vi "AE_continuousread.vi"() -> ()   [LabVIEW 2012]
doc: "I. Description:\nThis example demonstrates how to continuously acquire unscaled and save the data in a binary file. You can use the Graph Acquired Binary Data.VI to read and plot the scaled data on a Waveform Graph.\n\nII. Instructions for Running:\n1. Select the physical channel to correspond to where your signal is input on the DAQ device.\n2. Enter the minimum and maximum voltage ranges.\nNote: For better accuracy try to match the input range to the expected voltage level of the measured signal.\n3. Set the rate of the acquisition Also set the Samples to Read control. This will determine how many samples are read each time the while loop iterates. This also determines how many points are plotted on the graph each iteration.\nNote: The rate should be at least twice as fast as the maximum frequency component of the signal being acquired.\n4. Select the File Properties. If the file path is left empty, it will bring up a dialog box to let you browse to the file. \n\nIII. Block Diagram Steps:\n1. Create or replace a file to store the data.\n2. Create an analog input voltage channel.\n3. Set the rate for the sample clock. Additionally, define the sample mode to be continuous.\n4. Create a header and write it to the binary file.\n5. Call the Start VI to start acquiring samples. \n6. Read the unscaled data in a loop until the user hits the stop button or an error occurs.\nNote: This example uses unscaled I32 reads. Some devices support unscaled reads in smaller widths, such as I16. To get the maximum performance out of your device, use the unscaled read with the smallest supported width.\n7. Transpose the unscaled array of data and append it to the file.\n8. Close the File.\n9. Call the Stop VI to stop acquiring samples.\n10. Use the popup dialog box to display an error if any.\n\nIV. I/O Connections Overview:\nMake sure your signal input terminal matches the Physical Channel I/O control. For further connection information, refer to your hardware reference manual."
uses:
  <vilib>/Utility/error.llb/DialogType.ctl
  <vilib>/DAQmx/read.llb/DAQmx Read (Analog 1D Wfm NChan NSamp).vi
  <vilib>/DAQmx/create/channels.llb/DAQmx Create Channel (AI-Voltage-Basic).vi
  <vilib>/DAQmx/configure/timing.llb/DAQmx Timing (Sample Clock).vi
  Instance          10 57Saved   Cont Acq&Graph Voltage - Write Data to File (CSV) .vi
  <vilib>/DAQmx/miscellaneous.llb/DAQmx Fill In Error Info.vi
panel:
  in  "Gain":u16(ring)=1 items=["20 dB", "40 dB", "60 dB"]
  in  "Test Name":string="test"
  in  "Storage Directory":path=path "C:/Users/User/Desktop/Users_2013-2014/Michael Rossol"
  in  "stop":bool
  in  "Physical Channel":tag="Dev1/ai0"
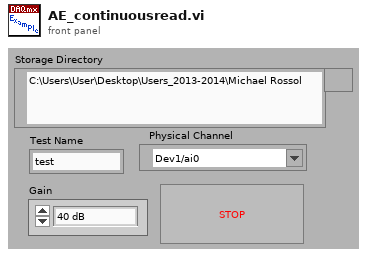
[diagram p1: front panel]
types:
  T1 = enum16{"open", "replace", "create", "open or create", "replace or create", "replace or create with confirmation"}
  T2 = typedef "DialogType.ctl" = u16
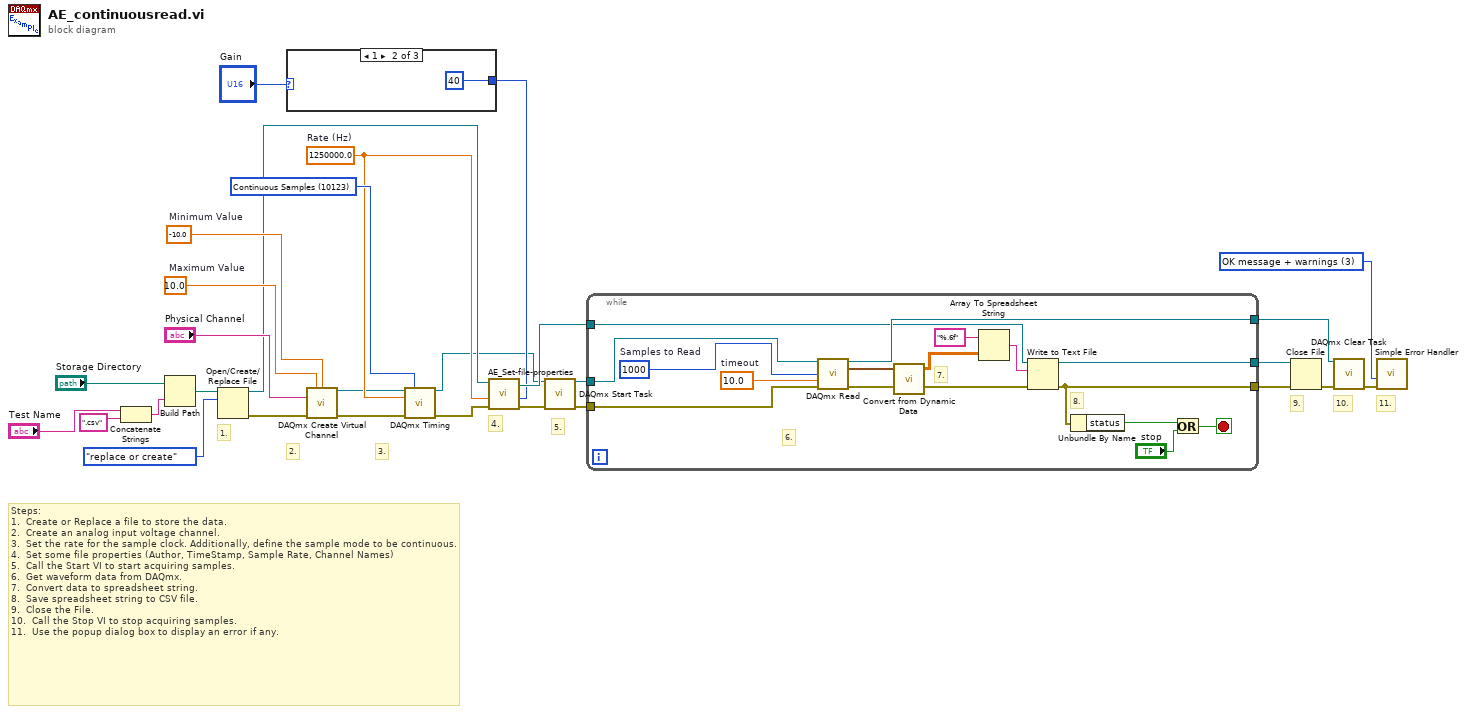
[diagram p0: block diagram]
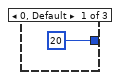
[diagram p2: hidden frame]
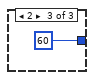
[diagram p3: hidden frame]
diagram:
  w13 = 1250000.0  # Rate (Hz)
  w28 = 10.0  # Maximum Value
  w29 = -10.0  # Minimum Value
  w19 = T2 3 items=["no dialog", "OK message", "continue or stop message", "OK message + warnings", "continue/stop + warnings"] ("type of dialog (OK msg:1)")
  w22 = 10123 items=["Finite Samples"=10178, "Continuous Samples"=10123] ("sample mode")
  # "11."
  # "10."
  # "4."
  # "9."
  # "3."
  # "5."
  # "Steps: \n1.  Create or Replace a file to store the data.\n2.  Create an analog input voltage channel.\n3.  Set the rate for the sample clock. Additionally, define the sample mode to be continuous.\n4.  Set some file properties (Author, TimeStamp, Sample Rate, Channel Names)\n5.  Call the Start VI to start acquiring samples.  \n6.  Get waveform data from DAQmx.\n7.  Convert data to spreadsheet string.\n8.  Save spreadsheet string to CSV file. \n9.  Close the File.\n10.  Call the Stop VI to stop acquiring samples.\n11.  Use the popup dialog box to display an error if any."
  # "2."
  # "1."
  n1 = Concatenate Strings("Test Name", ".csv" ("string")) -> (w6:string)
  n2 = Build Path(base path="Storage Directory", name or relative path=w6) -> (appended path=w4:path)
  n3 = Open/Create/Replace File(file path (use dialog)=w4, operation (0:open)=T1."replace or create") -> (refnum out=w10:refnum<file>, error out=w17:errorcluster)  [unwired: 4 in, 1 out]
  n4 = case shown="1" "Gain" {
    tunnel: [20 40 60] -> w2
    frame 0, Default {
    }
    frame 1 {
    }
    frame 2 {
    }
  }
  n5 = call-poly <vilib>:"DAQmx Create Virtual Channel.vi"("maximum value"=w28, "minimum value"=w29, "physical channels"="Physical Channel", "error in"=w17) -> ("task out"=w9:refnum<k21>, "error out"=w27:errorcluster)  [unwired: 10 in]
  n6 = call-poly <vilib>:"DAQmx Timing.vi"("task/channels in"=w9, "sample mode"=w22, "rate"=w13, "error in"=w27) -> ("task out"=w1:refnum<k21>, "error out"=w16:errorcluster)  [unwired: 10 in]
  n7 = call "AE_Set-file-properties.vi"("Gain (dB)"=w2, "error in (no error)"=w16, "Rate (Hz)"=w13, "text file"=w10) -> ("error out"=w15:errorcluster, "text file out"=w14:refnum<file>)  [unwired: 2 in]
  n8 = call <vilib>:"DAQmx Start Task.vi"("task/channels in"=w1, "error in"=w15) -> ("task out"=w25:refnum<k21>, "error out"=w26:errorcluster)  [unwired: 12 in]
  n9 = while {
    tunnel: w26 -> [w48]
    tunnel: w25 -> [w44]
    tunnel: [w43] -> w24
    tunnel: [w40] -> w21
    tunnel: [w39] -> w20
    tunnel: w14 -> [w37]
    stop <- w47 stop-if-true
    w41 = 1000  # Samples to Read
    w42 = 10.0  # timeout
    # "8."
    # "7."
    # "6."
    n10 = call-poly <vilib>:"DAQmx Read.vi"("task/channels in"=w44, "number of samples per channel"=w41, "timeout"=w42, "error in"=w48) -> ("task out"=w43:refnum<k21>, "data"=w33:waveform(dbl)[], "error out"=w38:errorcluster)  [unwired: 9 in]
    n11 = call "Convert from Dynamic Data"("Dynamic Data Type"=w33) -> ("Array"=w36:dbl[][])  [unwired: 3 in]
    n12 = Array To Spreadsheet String(array=w36, 3:"%.6f" ("format string")) -> (spreadsheet string=w34:string)  [unwired: 1 in]
    n13 = Write to Text File(file (use dialog)=w37, text=w34, error in=w38) -> (refnum out=w40:refnum<file>, error out=w39:errorcluster)  [unwired: 1 in, 1 out]
    n14 = Unbundle By Name(w39) -> ("status"=w45:bool)
    n15 = Or(x=w45, y="stop") -> (x .or. y?=w47:bool)
  }
  n16 = Close File(refnum=w21, error in=w20) -> (error out=w18:errorcluster)  [unwired: 1 out]
  n17 = call <vilib>:"DAQmx Clear Task.vi"("task in"=w24, "error in"=w18) -> ("error out"=w11:errorcluster)  [unwired: 13 in]
  n18 = call <vilib>:"Simple Error Handler.vi"("type of dialog (OK msg:1)"=w19, "error in (no error)"=w11) -> ()  [unwired: 3 in, 5 out]
